vi "plantita.vi"() -> ()   [LabVIEW 2015]
uses:
  Manual or Auto.ctl
  setpoints.ctl
  backwash.ctl
  coag.ctl
  model type.ctl
  data channels.ctl
  file paths.ctl
  state.ctl
  data ave state.ctl
  ini.ctl
  coagbuffer.ctl
  Sensor buffer command.ctl
  calcDoseorGetGraph.ctl
  <vilib>/addons/control/pid/pid.llb/PID (DBL).vi
  <vilib>/addons/control/pid/NI_PID_pid.lvlib
panel:
  in  "Tab Control":enum32{"Graphs", "Controls"}(tab)
  out "Misc":cluster{timestamp[], dbl[]}[](graph)
  out "Turbidities":cluster{timestamp[], dbl[]}[](graph)
  out "Coag Fitting Params":cluster{dbl[], "Best Linear Fit":dbl[]}[](graph)
  out "Sludge valve":dbl(graph)
  out "Coagulant [mg Al/L]":dbl(graph)
  out "Plant flow valve":dbl(graph)
  in  "data channel":T1
  in  "setpoints":T2={"graph data interval (s)"=100.0, "sludge flow [L/s]"=0.0, "plant flow [L/s]"=0.05, "Plant Flow PID "={"proportional gain (Kc)"=0.05, "integral time (Ti, min)"=1.0, "derivative time (Td, min)"=0.01}, "Sludge PID "={"proportional gain (Kc)"=0.07, "integral time (Ti, min)"=1.0, "derivative time (Td, min)"=0.01}, "backwash"={"Filtered quality target [NTU]"=0.3, "min filtration time [s]"=600.0, "Ripen time [s]"=600.0}, "Coagulant"={"flocculator volume (L)"=0.0, "clarifier volume (L)"=0.0, "dose updates per HRT"=100, "target clarified turbidity (NTU)"=0.3, "Coagulant mode"=enum."Manual", "Coag dose [mg/L]"=0.0}} {"Coagulant"."target clarified turbidity (NTU)" min=0.1 max=5.0 step=0.01; "Coagulant"."dose updates per HRT" min=1 max=1000 step=1; "Sludge PID"."derivative time (Td, min)" format="%.3f"; "Sludge PID"."integral time (Ti, min)" format="%.3f"; "Sludge PID"."proportional gain (Kc)" format="%.3f"; "Plant Flow PID"."derivative time (Td, min)" format="%.3f"; "Plant Flow PID"."integral time (Ti, min)" format="%.3f"; "Plant Flow PID"."proportional gain (Kc)" format="%.3f"; "plant flow [L/s]" min=0.05 max=1.0 step=0.05; "sludge flow [L/s]" min=0.0 max=0.05 step=0.001; "graph data interval (s)" min=1 max=1000 step=1}
  in  "Sludge valve [V]":dbl(slide)=1.5 scale=0.0..5.0
  in  "Sludge control":bool
  out "coag pump In Range?":bool
  out "coag model":T6
  in  "backwash [ON/OFF]":bool
  out "Last backwash":timestamp
  in  "Backwash control":T5
  out "error out":errorcluster
  out "total HRT":dbl
  out "recent data":dbl[](array[numeric])
  in  "channel":T1=enum."raw [NTU]"
  out "stopping":bool
  out "data labels":string[](array[string])
  in  "Shut Down":bool
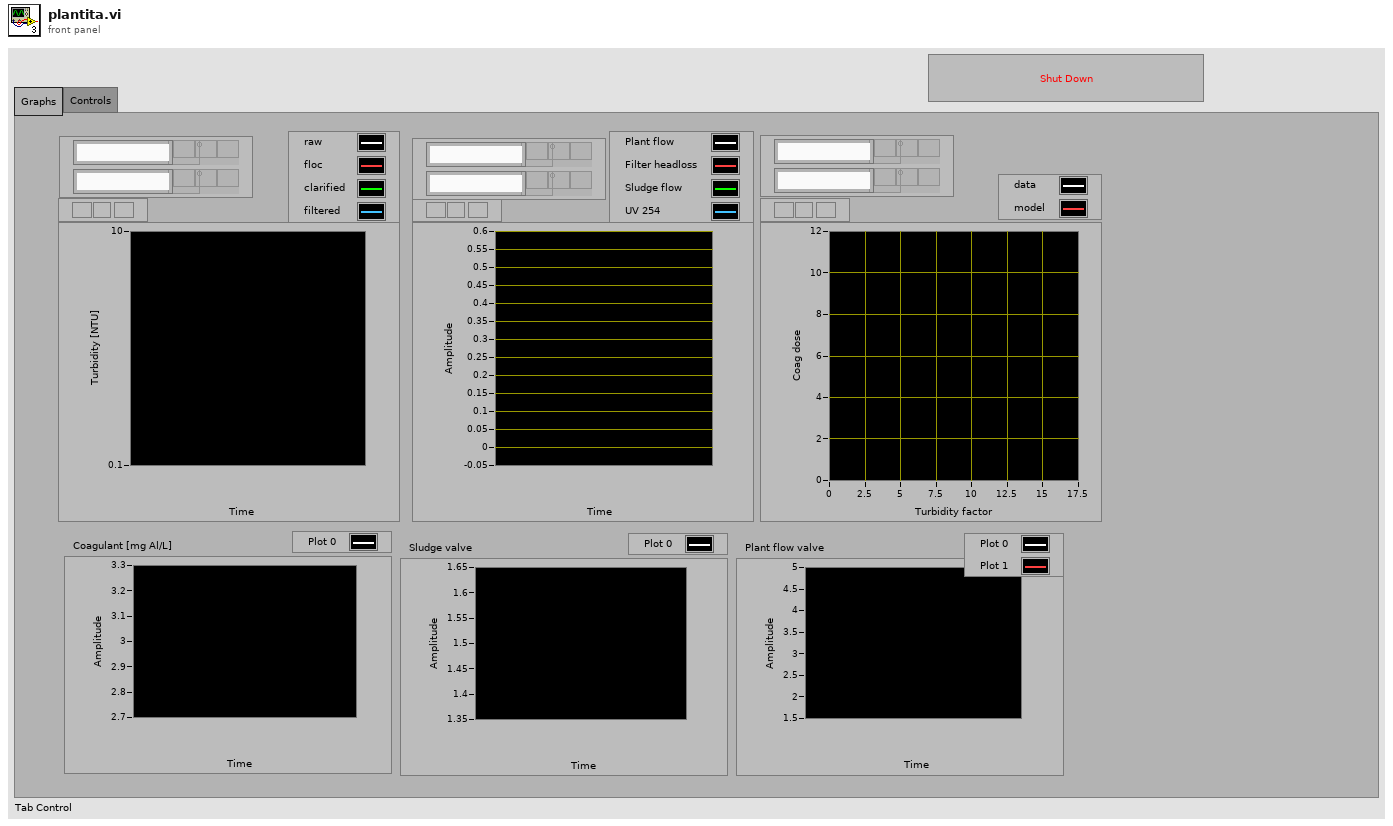
[diagram p1: front panel]
types:
  T1 = typedef "data channels.ctl" = enum16{"plant flow [L/s]", "Head Loss [m]", "sludge flow [L/s]", "UV 254", "raw [NTU]", "floc [NTU]", "clarified [NTU]", "filtered [NTU]"}
  T2 = typedef "setpoints.ctl" = cluster{"graph data interval (s)":sgl, "sludge flow [L/s]":dbl, "plant flow [L/s]":dbl, "Plant Flow PID ":cluster{"proportional gain (Kc)":dbl, "integral time (Ti, min)":dbl, "derivative time (Td, min)":dbl}, "Sludge PID ":cluster{"proportional gain (Kc)":dbl, "integral time (Ti, min)":dbl, "derivative time (Td, min)":dbl}, "backwash":T3, "Coagulant":T4}
  T3 = typedef "backwash.ctl" = cluster{"Filtered quality target [NTU]":dbl, "min filtration time [s]":dbl, "Ripen time [s]":dbl}
  T4 = typedef "coag.ctl" = cluster{"flocculator volume (L)":dbl, "clarifier volume (L)":dbl, "dose updates per HRT":u32, "target clarified turbidity (NTU)":dbl, "Coagulant mode":T5, "Coag dose [mg/L]":dbl}
  T5 = typedef "Manual or Auto.ctl" = enum16{"Manual", "Automatic"}
  T6 = typedef "model type.ctl" = enum16{"manual", "simple corrector", "linear regression"}
  T7 = typedef "file paths.ctl" = enum16{"read paths", "close"}
  T8 = typedef "ini.ctl" = enum16{"write", "read"}
  T9 = typedef "data ave state.ctl" = enum16{"Initialize", "Process data"}
  T10 = typedef "state.ctl" = enum16{"Initialize", "Process data", "Close"}
  T11 = typedef "coagbuffer.ctl" = enum16{"set buffer size", "write", "refill buffer", "read recent", "read all", "clear", "overwrite"}
  T12 = typedef "calcDoseorGetGraph.ctl" = enum16{"calculate dose", "read graph"}
  T13 = typedef "Sensor buffer command.ctl" = enum16{"set buffer size", "write", "refill buffer", "read recent", "read all", "clear"}
  T14 = cluster{"proportional gain (Kc)":dbl, "integral time (Ti, min)":dbl, "derivative time (Td, min)":dbl}
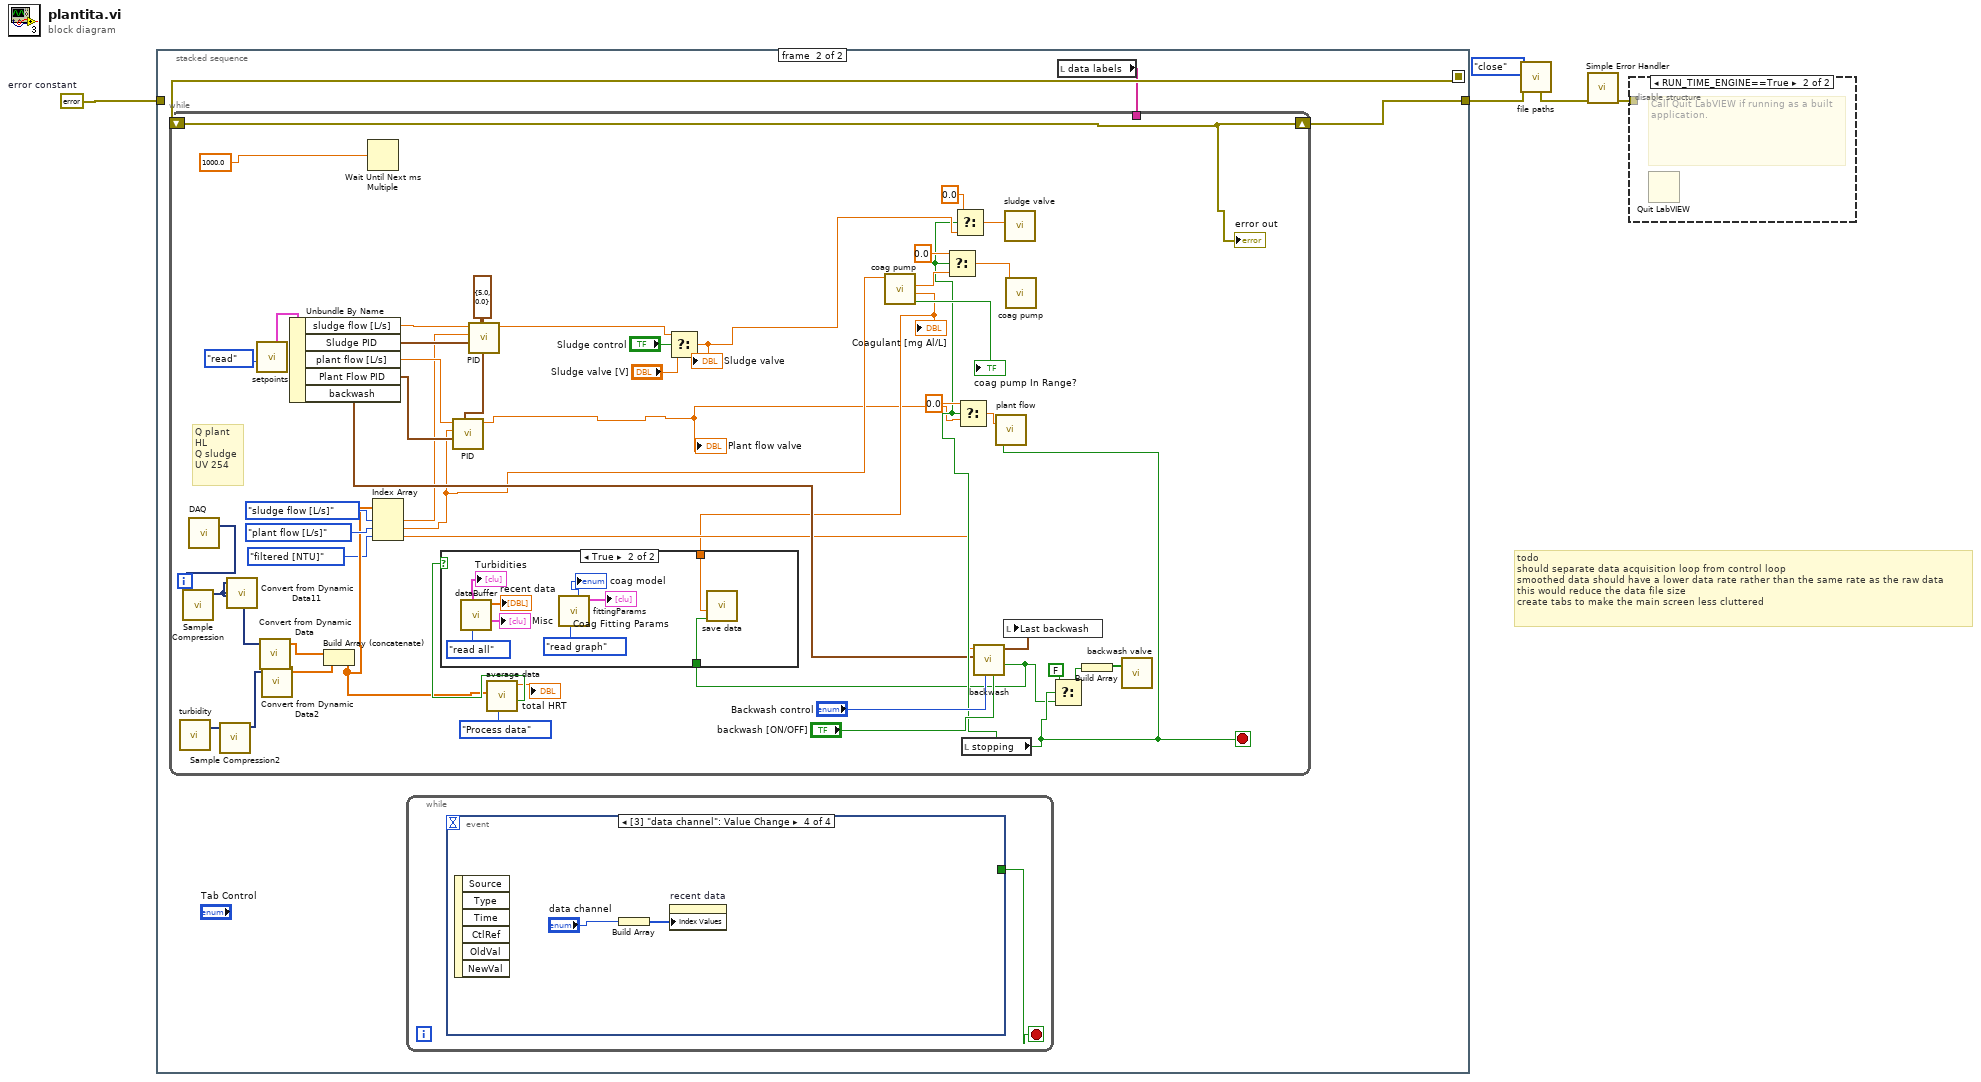
[diagram p0: block diagram]
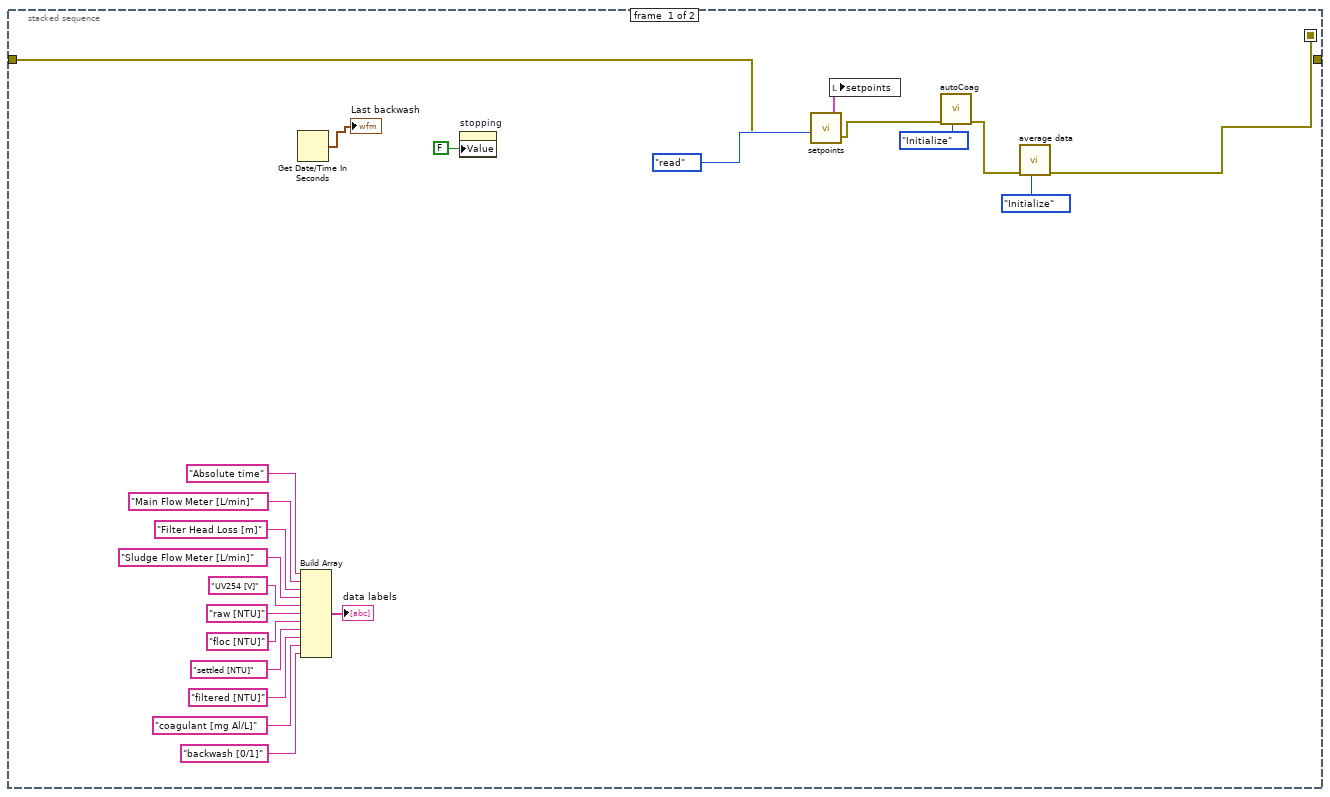
[diagram p2: hidden frame]
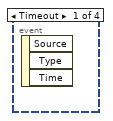
[diagram p3: hidden frame]
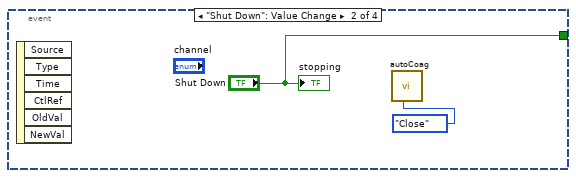
[diagram p4: hidden frame]
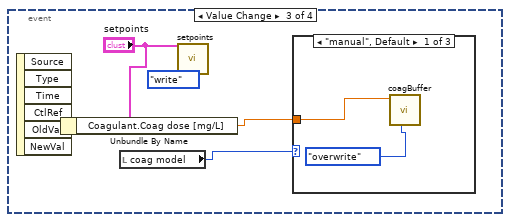
[diagram p5: hidden frame]
diagram:
  w5 = errorcluster {"status"=FALSE, "code"=0, "source"=""}  # error constant
  # "todo\nshould separate data acquisition loop from control loop\nsmoothed data should have a lower data rate rather than the same rate as the raw data\nthis would reduce the data file size\ncreate tabs to make the main screen less cluttered"
  n1 = stacked-sequence {
    seq-local: [w10 _] -> [_ w30]
    tunnel: w5 -> [w7 _]
    tunnel: [_ w28] -> w2
    frame #0 {
      n2 = Get Date/Time In Seconds() -> (seconds since 1Jan1904=→"Last backwash":timestamp)
      n3 = Build Array("Absolute time", "Main Flow Meter [L/min]", "Filter Head Loss [m]", "Sludge Flow Meter [L/min]", "UV254 [V]" ("element"), "raw [NTU]", "floc [NTU]", "settled [NTU]", "filtered [NTU]" ("element"), "coagulant [mg Al/L]" ("element"), "backwash [0/1]" ("element")) -> (→"data labels":string[])
      n4 = property on="stopping" class="Bool (strict)"("Value"=FALSE ("stopping")) -> ()  [unwired: 2 in, 2 out]
      n5 = call "setpoints.vi"("error in (no error)"=w7, "ini"=ini."read") -> ("error out"=w6:errorcluster, "Setpoints out"=w8:T2)  [unwired: 8 in]
      n6 = local write "setpoints"(w8) -> ()
      n7 = call "autoCoag.vi"("state"=state."Initialize" ("Enum"), "error in (no error)"=w6) -> ("error out"=w11:errorcluster)  [unwired: 7 in, 2 out]
      n8 = call "average data.vi"("state"=data_ave_state."Initialize", "error in (no error)"=w11) -> ("error out"=w10:errorcluster)  [unwired: 5 in, 4 out]
    }
    frame #1 {
      n9 = while {
        stop <- w31 stop-if-true
        n10 = event shown="[3] \"data channel\": Value Change" {
          selector: _ -> [_ _ _ _]
          dyn-events: _ -> [_ _ _ _]
          timeout: _ -> [_ _ _ _]
          tunnel: [_ "Shut Down" _ _] -> w31
          event Timeout {
            n11 = event-data() -> ()  [unwired: 1 in, 3 out]
          }
          event "Shut Down": Value Change {
            n12 = event-data() -> ()  [unwired: 1 in, 6 out]
            n13 = call "autoCoag.vi"("state"=state."Close" ("Enum")) -> ()  [unwired: 8 in, 3 out]
            "stopping" <- "Shut Down"
          }
          event Value Change {
            n14 = event-data() -> ()  [unwired: 1 in, 6 out]
            n15 = Unbundle By Name("setpoints") -> ("Coagulant.Coag dose [mg/L]"=w34:dbl)
            n16 = local read "coag model"() -> (w36:T6)
            n17 = call "setpoints.vi"("setpoints"="setpoints", "ini"=ini."write") -> ()  [unwired: 8 in, 2 out]
            n18 = case shown="\"manual\", Default" w36 {
              tunnel: w34 -> [w39 _ _]
              frame "manual", Default {
                n19 = call "coagBuffer.vi"("command"=coagbuffer."overwrite", "Coag dose"=w39) -> ()  [unwired: 7 in, 3 out]
              }
              frame "simple corrector" {
              }
              frame "linear regression" {
              }
            }
          }
          event Value Change {
            n20 = event-data() -> ()  [unwired: 1 in, 6 out]
            n21 = Build Array("data channel") -> (w40:T1[])
            n22 = property on="recent data" class="Arr (strict)"("Index Values"=w40) -> ()  [unwired: 2 in, 2 out]
          }
        }
      }
      n23 = local read "data labels"() -> (w29:string[])
      n24 = while {
        shift-right: [w54] -> w28
        shift-left: w30 -> [w54]
        tunnel: w29 -> [_]
        stop <- w71 stop-if-true
        w84 = cluster{"output high":dbl, "output low":dbl} {"output high"=5.0, "output low"=0.0} ("output range")
        # "Q plant\nHL\nQ sludge\nUV 254"
        n25 = call "turbidity"() -> ("data"=w57:dynamicdata)  [unwired: 17 in, 2 out]
        n26 = call "DAQ"() -> ("data"=w58:dynamicdata)  [unwired: 17 in, 2 out]
        n27 = call "Sample Compression"("Signals"=w58) -> ("Mean"=w53:dynamicdata)  [unwired: 8 in, 2 out]
        n28 = call "Sample Compression2"("Signals"=w57) -> ("Mean"=w48:dynamicdata)  [unwired: 8 in, 2 out]
        n29 = call "Convert from Dynamic Data11"("Dynamic Data Type"=w53) -> ()  [unwired: 3 in, 1 out]
        n30 = call "setpoints.vi"("ini"=ini."read") -> ("Setpoints out"=w55:T2)  [unwired: 9 in, 1 out]
        n31 = call "Convert from Dynamic Data"("Dynamic Data Type"=w53) -> ("Array"=w69:dbl[])  [unwired: 3 in]
        n32 = call "Convert from Dynamic Data2"("Dynamic Data Type"=w48) -> ("Array"=w68:dbl[])  [unwired: 3 in]
        n33 = Unbundle By Name(w55) -> ("sludge flow [L/s]"=w64:dbl, "Sludge PID"=w63:T14, "plant flow [L/s]"=w62:dbl, "Plant Flow PID"=w61:T14, "backwash"=w60:T3)
        n34 = Build Array (concatenate)(w69, w68) -> (w47:dbl[])
        n35 = Wait Until Next ms Multiple(millisecond multiple=1000.0 ("y")) -> ()  [unwired: 1 out]
        n36 = Index Array(array=w47, index #1=data_channels."sludge flow [L/s]" ("channel"), index #2=data_channels."plant flow [L/s]" ("channel"), index #3=data_channels."filtered [NTU]" ("channel")) -> (element #1=w50:dbl, element #2=w49:dbl, element #3=w45:dbl)
        n37 = call-poly <vilib>:"PID.vi"("output range"=w84, "PID gains"=w61, "process variable"=w49, "setpoint"=w62) -> ("output"=w42:dbl)  [unwired: 6 in, 1 out]
        "Plant flow valve" <- w42
        n38 = call-poly <vilib>:"PID.vi"("output range"=w84, "PID gains"=w63, "process variable"=w50, "setpoint"=w64) -> ("output"=w85:dbl)  [unwired: 6 in, 1 out]
        n39 = call "average data.vi"("state"=data_ave_state."Process data", "data input"=w47) -> ("new interval"=w65:bool, "total HRT"=→"total HRT":dbl)  [unwired: 5 in, 3 out]
        n40 = Select(t=w85, s="Sludge control", f="Sludge valve [V]") -> (s? t:f=w75:dbl)
        "Sludge valve" <- w75
        n41 = call "coag pump.vi"("plant flow [L/s]"=w49) -> ("In Range?"=→"coag pump In Range?":bool, "coag dose [mg/L]"=w44:dbl, "pump [V]"=w80:dbl)  [unwired: 7 in, 1 out]
        "Coagulant [mg Al/L]" <- w44
        n42 = local read "stopping"() -> (w71:bool)
        n43 = Select(t=0.0, s=w71, f=w80) -> (s? t:f=w79:dbl)
        n44 = Select(t=0.0, s=w71, f=w75) -> (s? t:f=w74:dbl)
        n45 = Select(t=0.0, s=w71, f=w42) -> (s? t:f=w78:dbl)
        n46 = call "backwash.vi"("Manual override"="backwash [ON/OFF]", "Backwash control"="Backwash control", "backwash"=w60, "Filtered Turbidity"=w45) -> ("backwashing?"=w43:bool, "last backwash"=w86:timestamp)  [unwired: 5 in, 1 out]
        n47 = case shown="True" w65 {
          tunnel: w44 -> [_ w93]
          tunnel: w43 -> [_ w92]
          frame False {
          }
          frame True {
            n48 = call "dataBuffer.vi"("command"=Sensor_buffer_command."read all") -> ("recent data"=→"recent data":dbl[], "misc graph"=→"Misc":cluster{timestamp[], dbl[]}[], "turbidity"=→"Turbidities":cluster{timestamp[], dbl[]}[])  [unwired: 5 in, 3 out]
            n49 = call "fittingParams.vi"("read/write"=calcDoseorGetGraph."read graph") -> ("Fitting Params"=→"Coag Fitting Params":cluster{dbl[], "Best Linear Fit":dbl[]}[], "coag model"=→"coag model":T6)  [unwired: 6 in, 3 out]
            n50 = call "save data.vi"("backwashing?"=w92, "coagulant dose"=w93) -> ()  [unwired: 10 in]
          }
        }
        n51 = call "plant flow"("data"=w78, "stop (T)"=w71) -> ()  [unwired: 16 in, 2 out]
        n52 = local write "Last backwash"(w86) -> ()
        n53 = call "sludge valve"("data"=w74) -> ()  [unwired: 17 in, 2 out]
        n54 = call "coag pump"("data"=w79) -> ()  [unwired: 17 in, 2 out]
        n55 = Select(t=FALSE, s=w71, f=w43) -> (s? t:f=w72:bool)
        n56 = Build Array(w72) -> (w89:bool[])
        n57 = call "backwash valve"("data"=w89) -> ()  [unwired: 17 in, 2 out]
        "error out" <- w54
      }
    }
  }
  n58 = call "file paths.vi"("error in (no error)"=w2, "file path control"=file_paths."close") -> ("error out"=w1:errorcluster)  [unwired: 6 in, 3 out]
  n59 = call <vilib>:"Simple Error Handler.vi"("error in (no error)"=w1) -> ("error out"=w4:errorcluster)  [unwired: 4 in, 4 out]
  n60 = disable-structure shown="RUN_TIME_ENGINE==True" {
    disable-tunnel: w4 -> [_ _]
    frame condition #0 (active) {
    }
    frame condition #1 {
      # "Call Quit LabVIEW if running as a built application."
      n61 = Quit LabVIEW() -> ()  [unwired: 1 in]
    }
  }
